vi "Camera.vi"() -> ()   [LabVIEW 2020]
uses:
  Control 1.ctl
panel:
  out "First Image 3":dbl[][](graph)
  out "Delta T":dbl[][][](array[numeric])
  out "subarray":dbl[][](array[numeric])
  out "FrameData 4":dbl[][][](array[numeric])
  out "FrameData 3":dbl[][][](array[numeric])
  out "Odd indices":i32[](array[numeric])
  out "even indices":i32[](array[numeric])
  out "FrameData":dbl[][][](array[numeric])
  out "ExtChData":dbl[][](array[numeric])
  in  "Timeout":i32
  in  "ExChs":i32
  in  "Frames":T1=1
  in  "Acq Trigger?":bool
  in  "Offset":i32=128 min=0 max=255 step=1
  out "Actual (us)":dbl
  in  "IntegrationTime (us)":dbl=0.1 min=0.1 max=5000.0 step=0.1
  out "MaxFrameRate":dbl
  in  "Frame Size (Row x Col)":u16(ring) items=["128x128", "96x128", "64x128", "32x128"]
  out "TempK":dbl
  out "First Image":dbl[][](graph)
  out "error":errorcluster
  # "IMAGE SETTINGS"
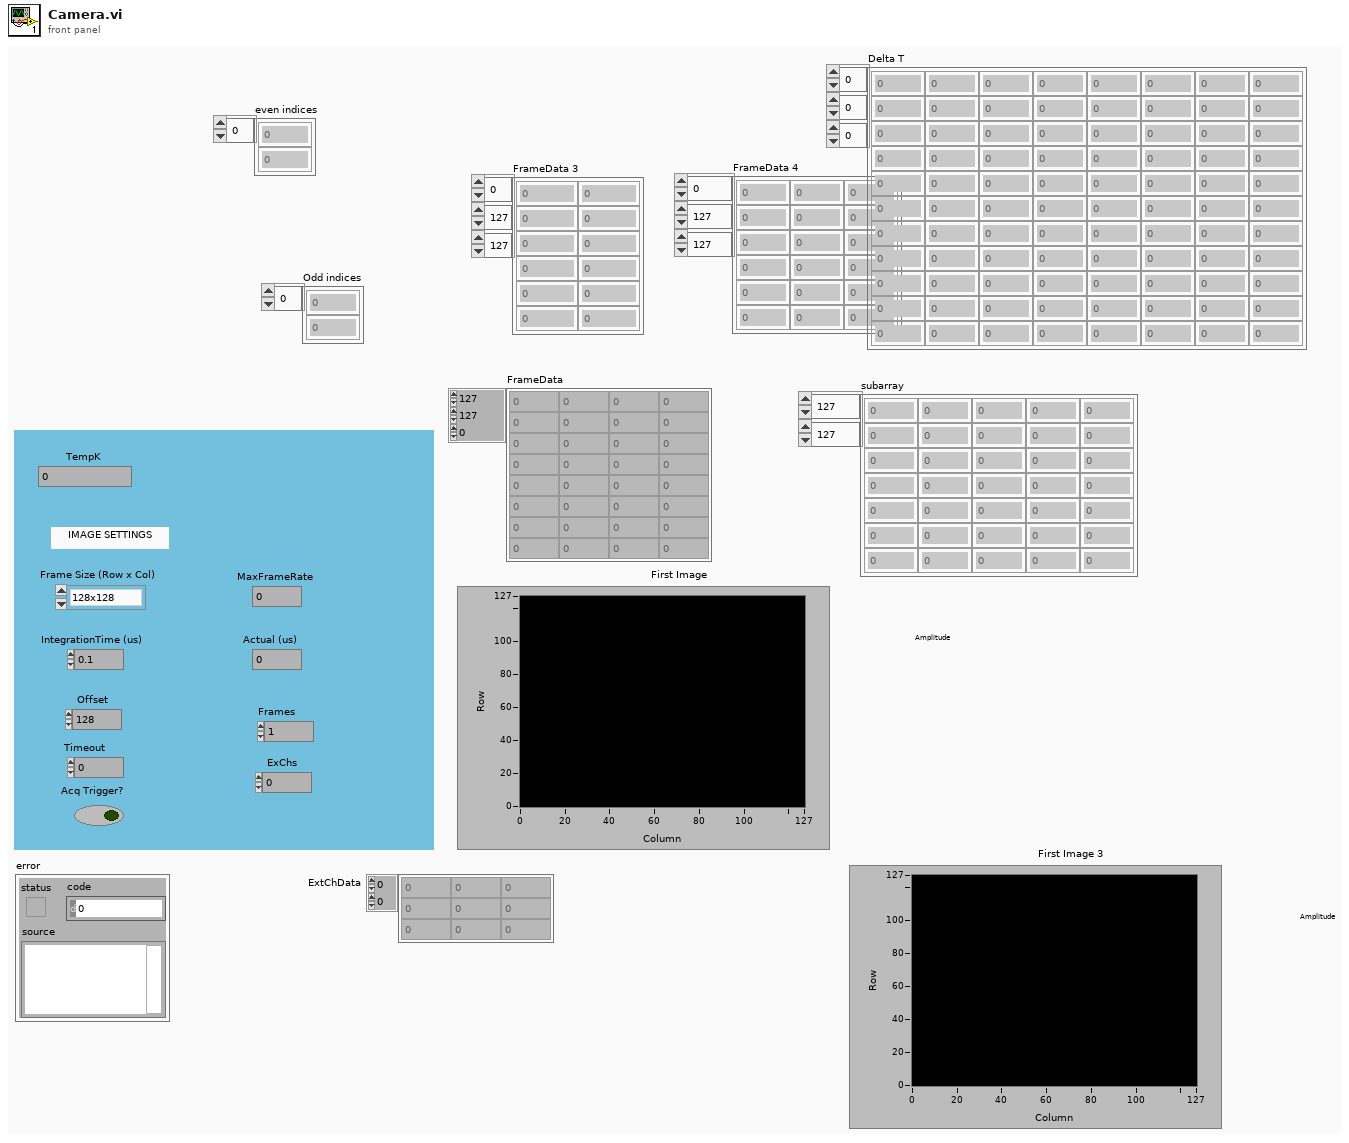
[diagram p1: front panel]
types:
  T1 = typedef "Control 1.ctl" = i32
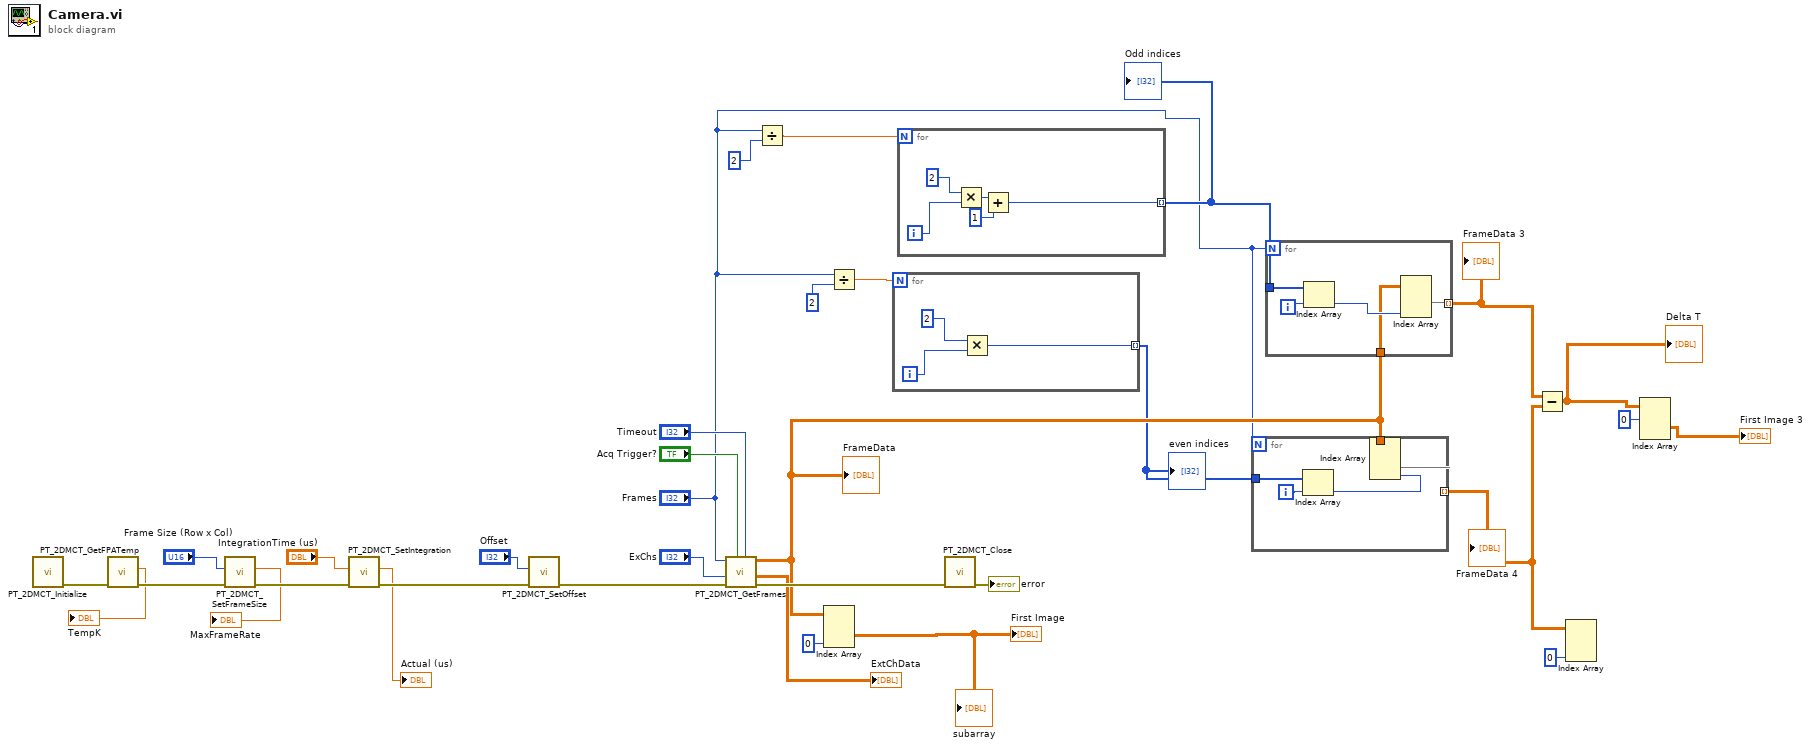
[diagram p0: block diagram]
diagram:
  n1 = call "PT_2DMCT_Initialize.vi"() -> ("error out"=w29:errorcluster)  [unwired: 11 in]
  n2 = call "PT_2DMCT_GetFPATemp.vi"("error in (no error)"=w29) -> ("error out"=w28:errorcluster, "TempK"=→"TempK":dbl)  [unwired: 8 in, 1 out]
  n3 = call "PT_2DMCT_SetFrameSize.vi"("error in (no error)"=w28, "Frame Size (Row x Col)"="Frame Size (Row x Col)") -> ("error out"=w27:errorcluster, "MaxFrameRate"=→"MaxFrameRate":dbl)  [unwired: 4 in]
  n4 = call "PT_2DMCT_SetIntegration.vi"("error in (no error)"=w27, "IntegrationTime (us)"="IntegrationTime (us)") -> ("error out"=w26:errorcluster, "Actual (us)"=→"Actual (us)":dbl)  [unwired: 4 in]
  n5 = call "PT_2DMCT_SetOffset.vi"("error in (no error)"=w26, "Offset"="Offset") -> ("error out"=w25:errorcluster)  [unwired: 9 in]
  n6 = call "PT_2DMCT_GetFrames.vi"("Timeout"="Timeout", "Acq Trigger?"="Acq Trigger?", "error in (no error)"=w25, "ExChs"="ExChs", "Frames"="Frames") -> ("error out"=w31:errorcluster, "ExtChData"=→"ExtChData":dbl[][], "FrameData"=w9:dbl[][][])  [unwired: 4 in]
  "FrameData" <- w9
  n7 = Divide(x="Frames", y=T1 2) -> (x/y=w11:dbl)
  n8 = Index Array(array=w9, index (dim 2)=0 ("disabled index (col)")) -> (element=→"First Image" →"subarray":dbl[][])  [unwired: 2 in]
  n9 = Divide(x="Frames", y=2) -> (x/y=w13:dbl)
  n10 = for {
    N: w13 -> [_]
    tunnel: [w34] -> w8 mode=indexing
    i -> [w36]
    n11 = Multiply(x=2, y=w36) -> (x*y=w34:i32)
  }
  "even indices" <- w8
  n12 = for {
    N: w11 -> [_]
    tunnel: [w37] -> w10 mode=indexing
    i -> [w41]
    n13 = Multiply(x=2, y=w41) -> (x*y=w39:i32)
    n14 = Add(x=w39, y=1) -> (x+y=w37:i32)
  }
  "Odd indices" <- w10
  n15 = call "PT_2DMCT_Close.vi"("error in (no error)"=w31) -> ("error out"=→"error":errorcluster)  [unwired: 10 in]
  n16 = for {
    N: "Frames" -> [_]
    tunnel: [w42] -> w4 mode=indexing
    tunnel: w9 -> [w44]
    tunnel: w8 -> [w45]
    i -> [w46]
    n17 = Index Array(array=w45, index=w46) -> (element=w43:i32)
    n18 = Index Array(array=w44, index (dim 2)=w43) -> (element=w42:dbl[][])  [unwired: 2 in]
  }
  "FrameData 4" <- w4
  n19 = for {
    N: "Frames" -> [_]
    tunnel: w10 -> [w51]
    tunnel: w9 -> [w48]
    tunnel: [w47] -> w6 mode=indexing
    i -> [w50]
    n20 = Index Array(array=w51, index=w50) -> (element=w49:i32)
    n21 = Index Array(array=w48, index (dim 2)=w49) -> (element=w47:dbl[][])  [unwired: 2 in]
  }
  "FrameData 3" <- w6
  n22 = Subtract(x=w6, y=w4) -> (x-y=w3:dbl[][][])
  "Delta T" <- w3
  n23 = Index Array(array=w4, index (dim 2)=0 ("disabled index (col)")) -> ()  [unwired: 2 in, 1 out]
  n24 = Index Array(array=w3, index (dim 0)=0 ("index (page)")) -> (element=→"First Image 3":dbl[][])  [unwired: 2 in]
